vi "Untitled 1, Aula 4 (João).vi"() -> ()   [LabVIEW 2024]
uses:
  <vilib>/numeric/Random Number (Range) DBL.vi
panel:
  out "Tensão fase C":dbl[](array[numeric])
  out "Corrente fase C":dbl[](array[numeric])
  out "Potencia ativa":dbl[](array[numeric])
  out "Potencia ativa C":dbl[](graph)
  out "Fator portencia 3":dbl
  in  "Limite inferior FP 3":dbl
  in  "Limite superior FP 3":dbl=100.0
  out "Corrente fase B":dbl[](array[numeric])
  out "Tensão fase B":dbl[](array[numeric])
  out "Potencia ativa B":dbl[](array[numeric])
  out "Potencia ativa B":dbl[](graph)
  out "Fator portencia 2":dbl
  in  "Limite inferior FP 2":dbl
  in  "Limite superior FP 2":dbl=100.0
  out "Potencia ativa A":dbl[](array[numeric])
  out "Fator portencia":dbl
  out "Corrente fase A":dbl[](array[numeric])
  out "Tensão fase A":dbl[](array[numeric])
  in  "Limite inferior FP":dbl
  in  "Limite superior FP":dbl=100.0
  out "Potencia ativa A":dbl[](graph)
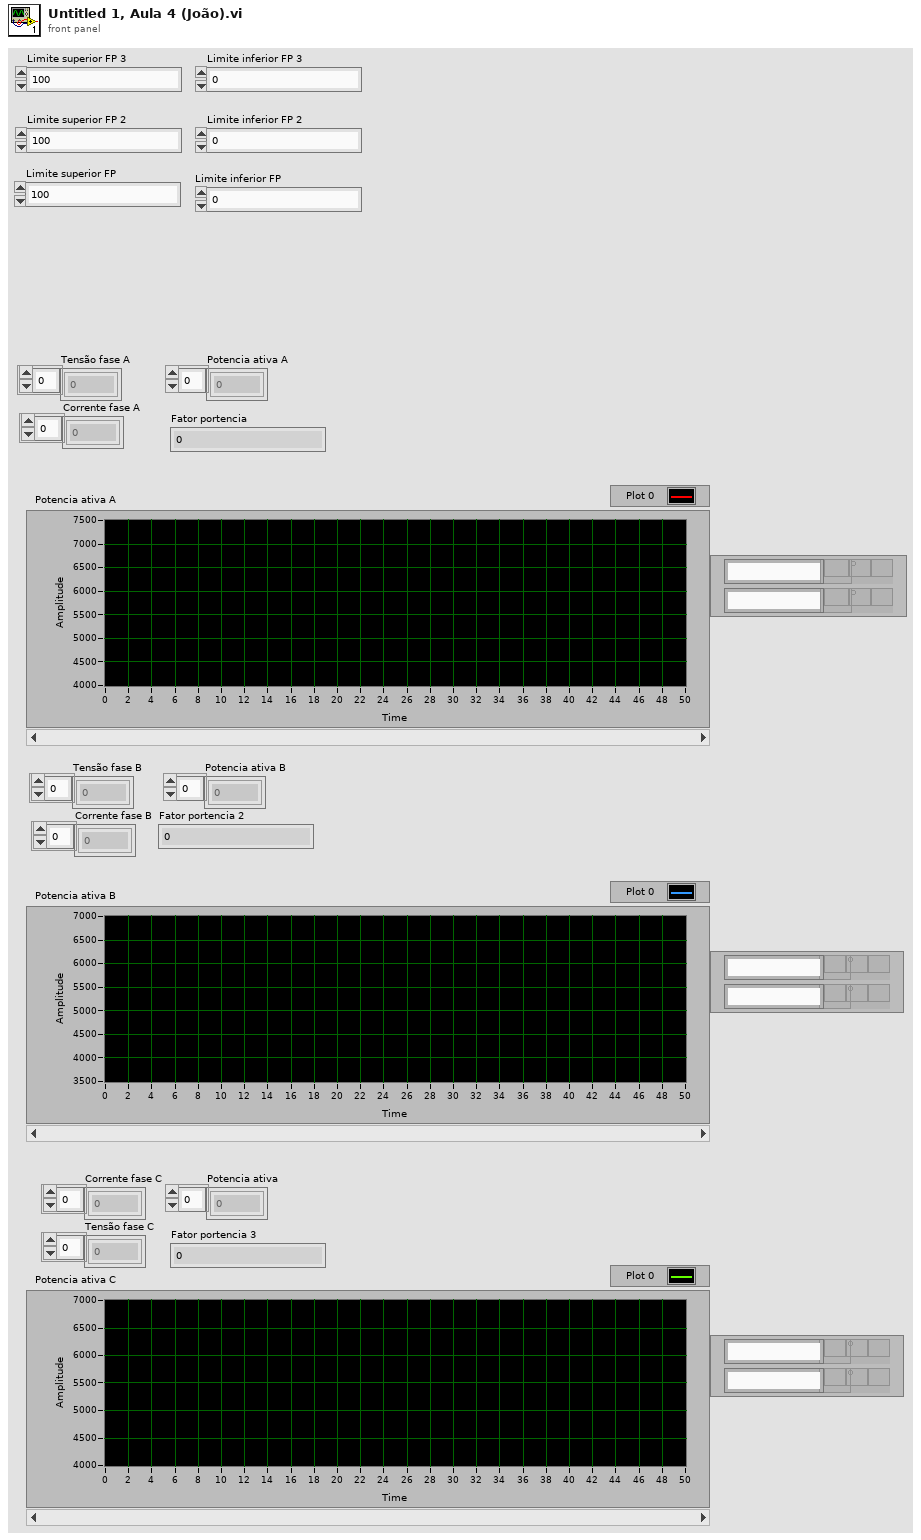
[diagram p1: front panel]
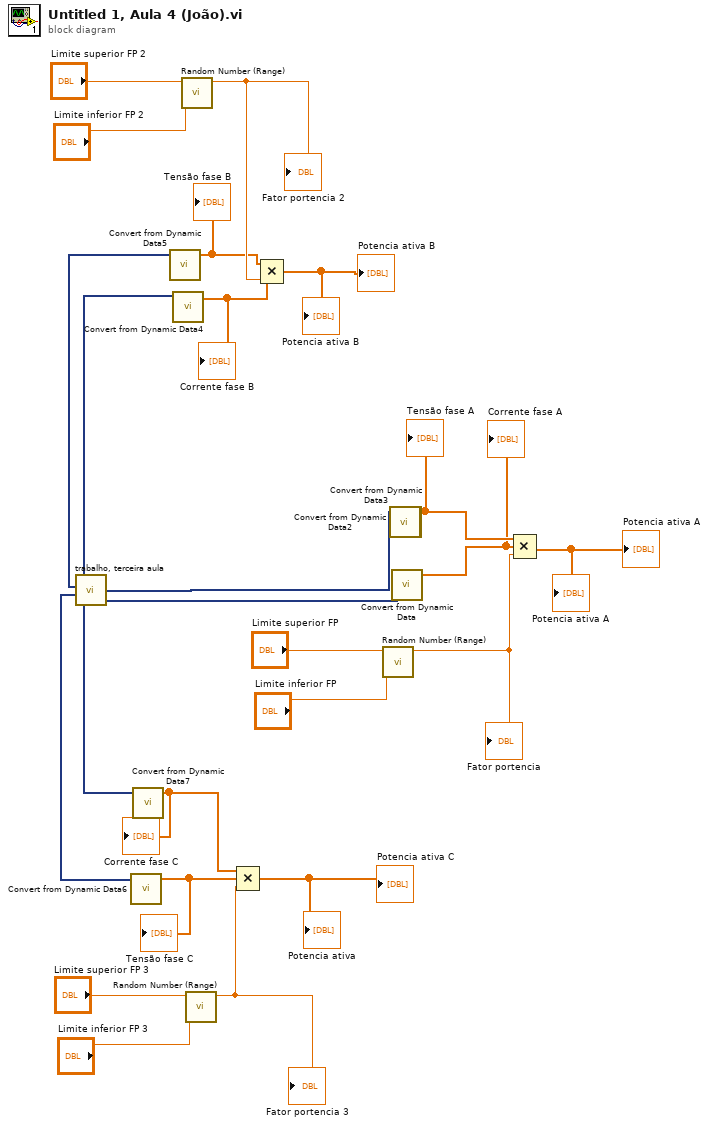
[diagram p0: block diagram]
diagram:
  n1 = call "trabalho, terceira aula.vi"() -> ("Corrente fase A"=w21:dynamicdata, "Tensão fase A"=w22:dynamicdata, "Corrente fase C"=w7:dynamicdata, "Tensão fase C"=w8:dynamicdata, "Corrente fase B"=w15:dynamicdata, "Tensão fase B"=w16:dynamicdata)  [unwired: 1 out]
  n2 = call "Convert from Dynamic Data6"("Dynamic Data Type"=w8) -> ("Array"=w1:dbl[])  [unwired: 3 in]
  "Tensão fase C" <- w1
  n3 = call "Convert from Dynamic Data7"("Dynamic Data Type"=w7) -> ("Array"=w2:dbl[])  [unwired: 3 in]
  "Corrente fase C" <- w2
  n4 = call "Convert from Dynamic Data5"("Dynamic Data Type"=w15) -> ("Array"=w10:dbl[])  [unwired: 3 in]
  "Tensão fase B" <- w10
  n5 = call "Convert from Dynamic Data4"("Dynamic Data Type"=w16) -> ("Array"=w9:dbl[])  [unwired: 3 in]
  "Corrente fase B" <- w9
  n6 = call-poly <vilib>:"Random Number (Range).vi"("lower bound (0)"="Limite inferior FP 2", "upper bound (100)"="Limite superior FP 2") -> ("number"=w12:dbl)  [unwired: 9 in]
  "Fator portencia 2" <- w12
  n7 = call-poly <vilib>:"Random Number (Range).vi"("lower bound (0)"="Limite inferior FP 3", "upper bound (100)"="Limite superior FP 3") -> ("number"=w4:dbl)  [unwired: 9 in]
  "Fator portencia 3" <- w4
  n8 = Compound Arithmetic op=MULTIPLY(w2, w1, w4) -> (→"Potencia ativa C" →"Potencia ativa":dbl[])
  n9 = Compound Arithmetic op=MULTIPLY(w10, w9, w12) -> (→"Potencia ativa B" →"Potencia ativa B":dbl[])
  n10 = call-poly <vilib>:"Random Number (Range).vi"("lower bound (0)"="Limite inferior FP", "upper bound (100)"="Limite superior FP") -> ("number"=w18:dbl)  [unwired: 9 in]
  "Fator portencia" <- w18
  n11 = call "Convert from Dynamic Data2"("Dynamic Data Type"=w22) -> ("Array"=w20:dbl[])  [unwired: 3 in]
  "Tensão fase A" <- w20
  n12 = call "Convert from Dynamic Data3"() -> ()  [unwired: 4 in, 1 out]
  n13 = call "Convert from Dynamic Data"("Dynamic Data Type"=w21) -> ("Array"=w19:dbl[])  [unwired: 3 in]
  "Corrente fase A" <- w19
  n14 = Compound Arithmetic op=MULTIPLY(w20, w19, w18) -> (→"Potencia ativa A" →"Potencia ativa A":dbl[])
